vi "Get All Channels.vi"(8 "error in (no error)":errorcluster, 11 "VISA Refnum in":refnum<visa-resource-name>="COM1") -> (0 "error out":errorcluster, 2 "allChannelProperties":T1 {"channel" min=1 max=8 step=1}, 3 "VISA Refnum out":refnum<visa-resource-name>)   [LabVIEW 2019, in "KH7008.lvlib"]
uses:
  KH7008.lvlib
  typedefs/allChannelProperties--Array.ctl
  typedefs/channelProperties--Cluster.ctl
  typedefs/channel--numeric.ctl
  typedefs/gain--enum.ctl
  typedefs/Input--Enum.ctl
  typedefs/shunt--enum.ctl
  typedefs/couple--Enum.ctl
  typedefs/Filter--Enum.ctl
  bfe76388-2f53-48f9-a091-37d1265c9076.vi
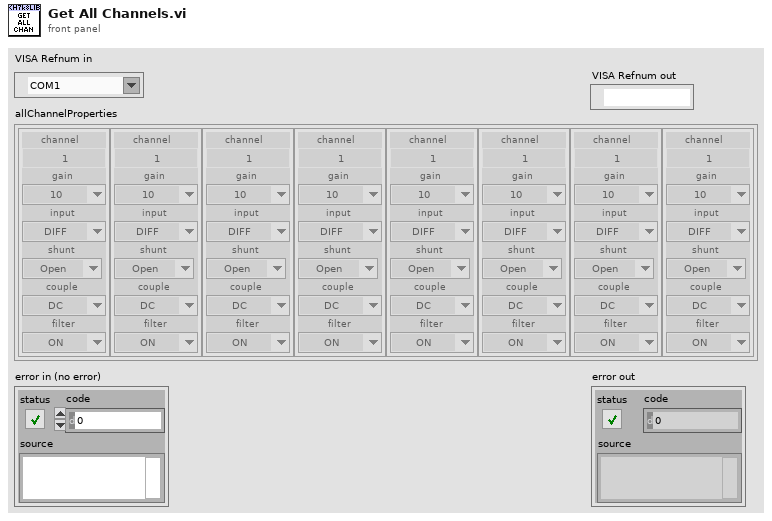
[diagram p1: front panel]
types:
  T1 = typedef "KH7008.lvlib/allChannelProperties--Array.ctl" = T2[]
  T2 = typedef "KH7008.lvlib/channelProperties--Cluster.ctl" = cluster{"channel":T3, "gain":T4, "input":T5, "shunt":T6, "couple":T7, "filter":T8}
  T3 = typedef "KH7008.lvlib/channel--numeric.ctl" = u16
  T4 = typedef "KH7008.lvlib/gain--enum.ctl" = enum16{"1", "10", "100", "1000"}
  T5 = typedef "KH7008.lvlib/input--enum.ctl" = enum16{"OFF", "SE+", "SE-", "DIFF"}
  T6 = typedef "KH7008.lvlib/shunt--enum.ctl" = enum16{"Open", "50", "500", "5k", "50k", "10M"}
  T7 = typedef "KH7008.lvlib/couple--enum.ctl" = enum16{"AC", "DC"}
  T8 = typedef "KH7008.lvlib/filter--enum.ctl" = enum16{"OFF", "ON"}
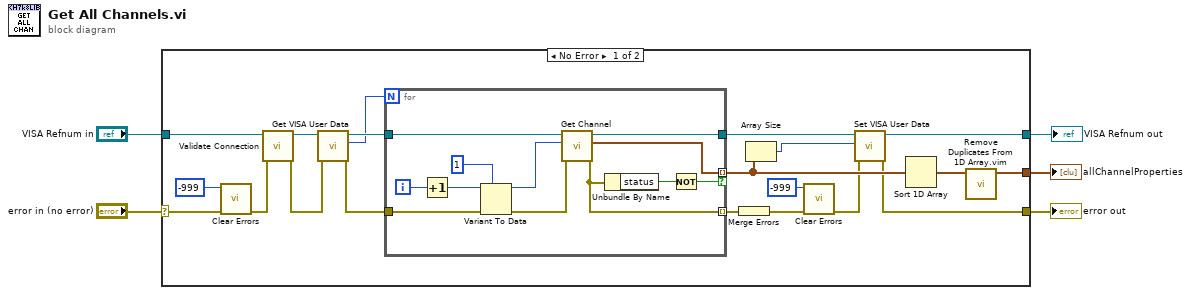
[diagram p0: block diagram]
diagram:
  n1 = case shown="No Error" "error in (no error)" {
    selector: "error in (no error)" -> [w25 w39]
    tunnel: "VISA Refnum in" -> [w10 w38]
    tunnel: [w17 w38] -> w4
    tunnel: [w11 w39] -> w2
    tunnel: [w6 _] -> w1
    frame No Error {
      n2 = call <vilib>:"Clear Errors.vi"("error in (no error)"=w25, "specific error code to clear (0: all)"=-999) -> ("error out"=w9:errorcluster)  [unwired: 4 in, 1 out]
      n3 = call "Validate Connection.vi"("error in (no error)"=w9, "VISA Refnum in"=w10) -> ("error out"=w7:errorcluster, "VISA Refnum out"=w8:refnum<visa-resource-name>)  [unwired: 8 in]
      n4 = call "Get VISA User Data.vi"("error in (no error)"=w7, "VISA Refnum in"=w8) -> ("error out"=w16:errorcluster, "User Data"=w14:i32, "VISA Refnum out"=w15:refnum<visa-resource-name>)  [unwired: 7 in]
      n5 = for {
        N: w14 -> [_]
        tunnel: w15 -> [w37]
        tunnel: [w36] -> w18
        tunnel: w16 -> [w32]
        tunnel: [w29] -> w22 mode=indexing
        tunnel: [w26] -> w20 mode=indexing if=w28
        i -> [w34]
        n6 = Increment(x=w34) -> (x+1=w27:i32)
        n7 = Variant To Data(error in=w32, type=T3 1 ("Channel"), Variant=w27) -> (data=w31:T3, error out=w33:errorcluster)
        n8 = call "Get Channel.vi"("error in (no error)"=w33, "channel"=w31, "VISA Refnum in"=w37) -> ("error out"=w29:errorcluster, "channelProperties"=w26:T2, "VISA Refnum out"=w36:refnum<visa-resource-name>)  [unwired: 6 in]
        n9 = Unbundle By Name(w29) -> ("status"=w30:bool)
        n10 = Not(x=w30) -> (.not. x?=w28:bool)
      }
      n11 = Merge Errors(w22) -> (w13:errorcluster)
      n12 = Array Size(array=w20) -> (size(s)=w19:i32)
      n13 = call <vilib>:"Clear Errors.vi"("error in (no error)"=w13, "specific error code to clear (0: all)"=-999) -> ("error out"=w12:errorcluster)  [unwired: 4 in, 1 out]
      n14 = call "Set VISA User Data.vi"("error in (no error)"=w12, "User Data"=w19, "VISA Refnum in"=w18) -> ("error out"=w11:errorcluster, "VISA Refnum out"=w17:refnum<visa-resource-name>)  [unwired: 7 in]
      n15 = Sort 1D Array(array=w20) -> (sorted array=w21:T2[])
      n16 = call "Remove Duplicates From 1D Array.vim"("array"=w21) -> ("array with duplicates removed"=w6:T2[])  [unwired: 10 in]
    }
    frame Error {
    }
  }
  "error out" <- w2
  "VISA Refnum out" <- w4
  "allChannelProperties" <- w1
